vi "FTW-Endpoint-Bind.vi"(0 "FTW Endpoint":refnum<class "FTW-Endpoint-TCP.lvclass">, 5 "Endpoint Address":string, 7 "Requested Identity":string, 11 "error in":errorcluster) -> (4 "FTW Endpoint out":refnum<class "FTW-Endpoint-TCP.lvclass">, 6 "Actual Endpoint Address":string, 8 "Actual Identity":string, 15 "error out":errorcluster)   [LabVIEW 2013, in "FTW-Endpoint-TCP.lvclass"]
uses:
  FTW-Endpoint-TCP.lvclass
  FTW-Endpoint-TCP.lvclass/FTW-Endpoint-TCP.ctl
panel:
  # "Inputs"
  # "Outputs"
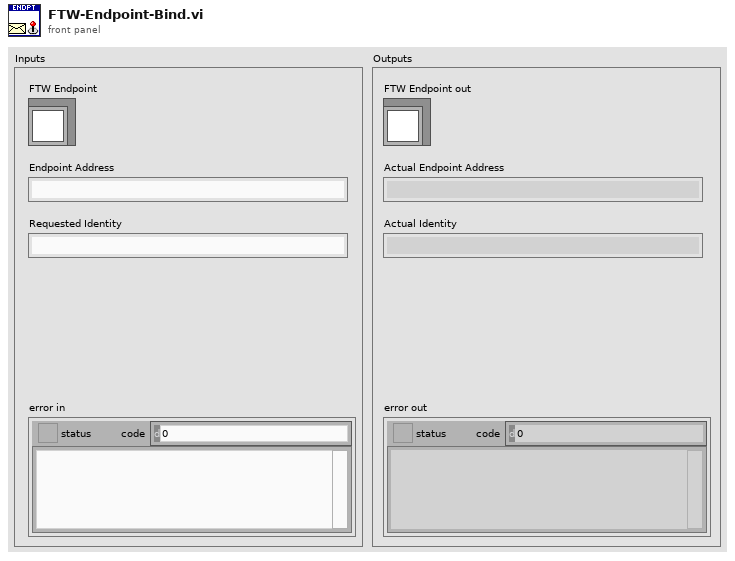
[diagram p1: front panel]
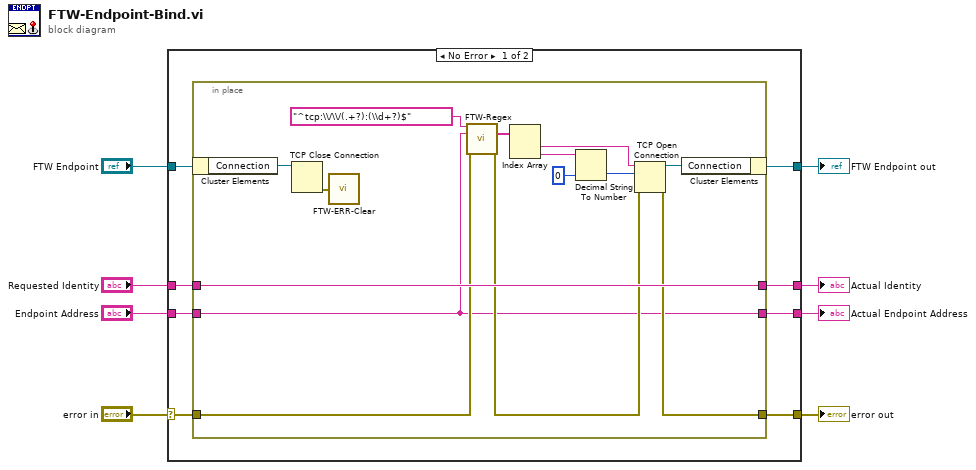
[diagram p0: block diagram]
diagram:
  n1 = case shown="No Error" "error in" {
    selector: "error in" -> [w14 w32]
    tunnel: [w10 w32] -> w8
    tunnel: [w11 w31] -> w6
    tunnel: "FTW Endpoint" -> [w16 w31]
    tunnel: "Requested Identity" -> [w15 _]
    tunnel: "Endpoint Address" -> [w13 _]
    tunnel: [w12 _] -> w2
    tunnel: [w9 _] -> w1
    frame No Error {
      n2 = in-place {
        in-place-border: w15 -> [w29]
        in-place-border: w14 -> [w19]
        in-place-border: [w22] -> w10
        in-place-border: w13 -> [w17]
        in-place-border: [w17] -> w12
        in-place-border: [w29] -> w9
        n3 = in-place-cluster #1(w16) -> ("Connection"=w30:refnum<k5>)
        n4 = TCP Close Connection(connection ID=w30) -> (error out=w25:errorcluster)  [unwired: 2 in, 1 out]
        n5 = call "FTW-ERR-Clear.vi"("error to snuff"=w25) -> ()  [unwired: 1 out]
        n6 = call "FTW-Regex.vi"("Regular Expression"="^tcp:\\/\\/(.+?):(\\d+?)$" ("input string"), "Input String"=w17, "error in"=w19) -> ("Submatches"=w28:string[], "error out"=w18:errorcluster)  [unwired: 8 in, 3 out]
        n7 = Index Array(array=w28) -> (element #1=w21:string, element #2=w27:string)  [unwired: 2 in]
        n8 = Decimal String To Number(string=w27, default (0L)=u16 0 ("remote port or service name")) -> (number=w20:u16)  [unwired: 1 in, 1 out]
        n9 = TCP Open Connection(address=w21, remote port or service name=w20, error in (no error)=w18) -> (connection ID=w23:refnum<k5>, error out=w22:errorcluster)  [unwired: 2 in]
        n10 = in-place-cluster #1("Connection"=w23) -> (w11:refnum<class "FTW-Endpoint-TCP.lvclass">)
      }
    }
    frame Error {
    }
  }
  "error out" <- w8
  "FTW Endpoint out" <- w6
  "Actual Endpoint Address" <- w2
  "Actual Identity" <- w1
